vi "bylinear interpolation iiii- complex.vi"(0 "Array":cdb[](array[numeric]), 11 "center":i32=-1) -> (1 "radius":dbl, 2 "sigma":dbl, 3 "directed sigma - abs":dbl, 4 "left":cdb, 6 "center":cdb, 8 "right":cdb, 10 "directed sigma":cdb, 12 "intercept":cdb, 13 "slope":cdb, 14 "curvature":cdb, 15 "circle center":cdb)   [LabVIEW 2020]
uses:
  <vilib>/Analysis/baseanly.llb/Complex A x B.vi
  Q - not nan -- real.vi
  <vilib>/Analysis/Matrix/Numeric/Conversions/Array To Matrix.vi
  <vilib>/Analysis/Matrix/Numeric/Conversions/Array To Matrix - RA2.vi
  <vilib>/Analysis/baseanly.llb/Inverse Matrix.vi
  <vilib>/Analysis/baseanly.llb/Real Inverse Matrix.vi
  <vilib>/Analysis/NI_AALBase.lvlib
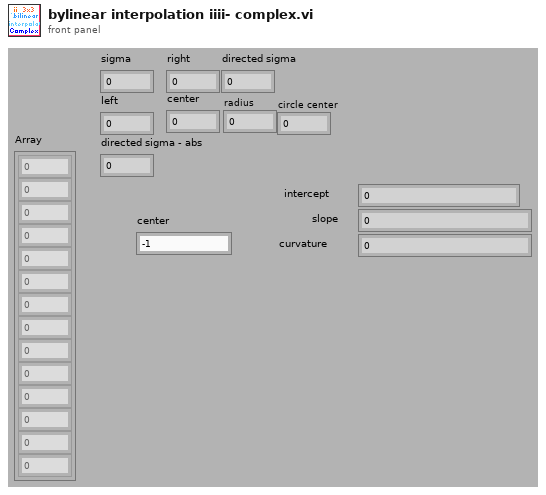
[diagram p1: front panel]
types:
  T1 = typedef "NI_Matrix.lvlib/RealMatrix.ctl" = dbl[][]
  T2 = typedef "NI_Matrix.lvlib/ComplexMatrix.ctl" = cdb[][]
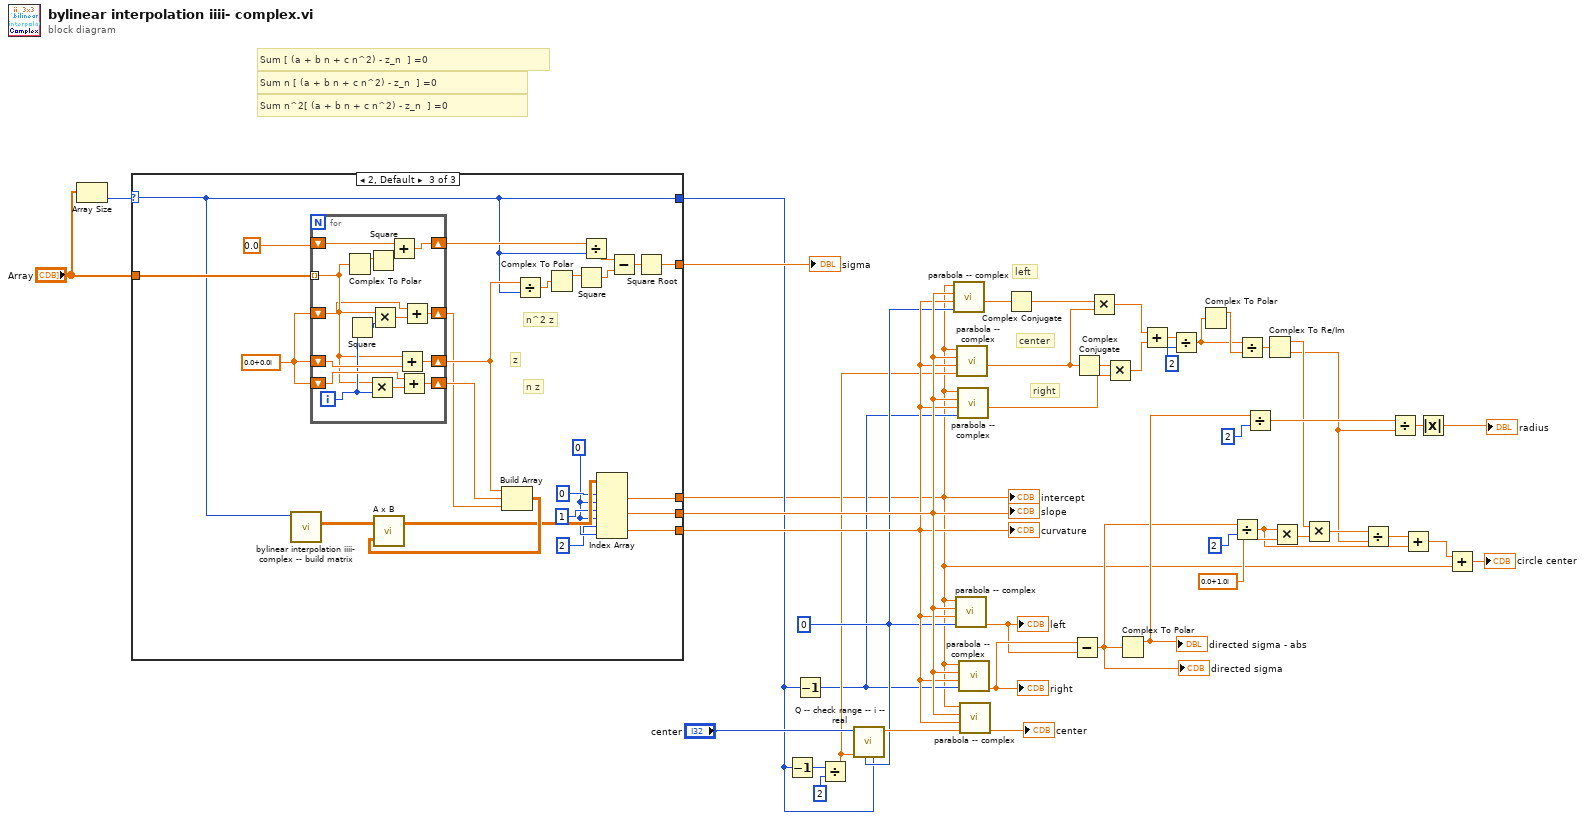
[diagram p0: block diagram]
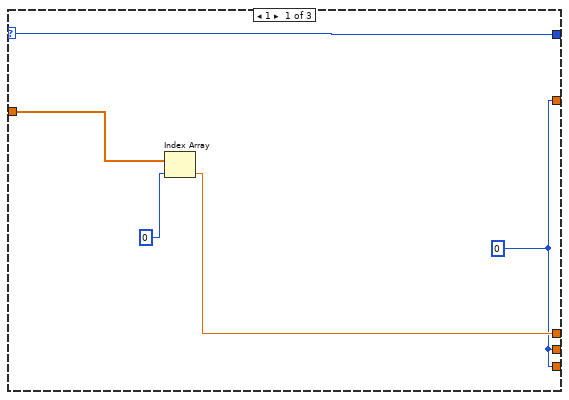
[diagram p2: hidden frame]
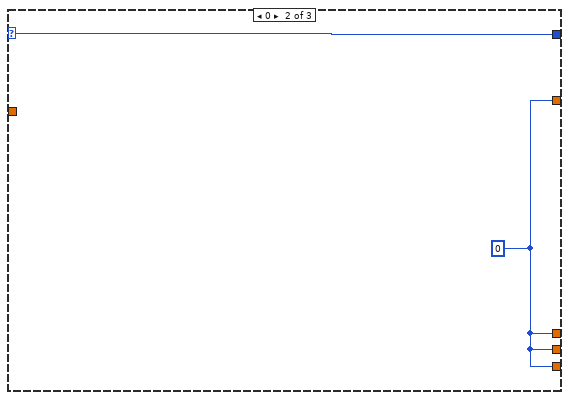
[diagram p3: hidden frame]
diagram:
  w35 = 0 ("n")
  # "right"
  # "center"
  # "left"
  # "Sum n^2[ (a + b n + c n^2) - z_n  ] =0"
  # "Sum n [ (a + b n + c n^2) - z_n  ] =0"
  # "Sum [ (a + b n + c n^2) - z_n  ] =0"
  n1 = Array Size(array="Array") -> (size(s)=w4:i32)
  n2 = case shown="2, Default" w4 {
    selector: w4 -> [w47 w52 w53]
    tunnel: [w48 w51 w56] -> w10
    tunnel: [w46 w51 w55] -> w37
    tunnel: "Array" -> [w50 _ w76]
    tunnel: [w46 w51 w75] -> w45
    tunnel: [w47 w52 w53] -> w33
    tunnel: [w46 w51 w54] -> w36
    frame 1 {
      w46 = 0 ("index")
      n3 = Index Array(array=w50, index=0) -> (element=w48:cdb)
    }
    frame 0 {
      w51 = 0 ("index")
    }
    frame 2, Default {
      w58 = 0 ("index (row)")
      w67 = cdb 0.0+0.0i
      # "n z"
      # "z"
      # "n^2 z"
      n4 = call "bylinear interpolation iiii- complex -- build matrix.vi"("N"=w53) -> ("Inverse Matrix"=w63:T1)  [unwired: 10 in]
      n5 = for {
        tunnel: w76 -> [w79] mode=indexing
        shift-right: [w91] -> w66
        shift-left: w67 -> [w90]
        shift-right: [w88] -> w65
        shift-left: w67 -> [w87]
        shift-right: [w86] -> w74
        shift-left: 0.0 -> [w85]
        shift-right: [w78] -> w64
        shift-left: w67 -> [w77]
        i -> [w82]
        n6 = Complex To Polar(r * e^(i*theta)=w79) -> (r=w84:dbl)  [unwired: 1 out]
        n7 = Square(x=w82) -> (x^2=w80:i32)
        n8 = Multiply(x=w79, y=w82) -> (x*y=w89:cdb)
        n9 = Square(x=w84) -> (x^2=w83:dbl)
        n10 = Multiply(x=w79, y=w80) -> (x*y=w81:cdb)
        n11 = Add(x=w85, y=w83) -> (x+y=w86:dbl)
        n12 = Add(x=w79, y=w90) -> (x+y=w91:cdb)
        n13 = Add(x=w87, y=w89) -> (x+y=w88:cdb)
        n14 = Add(x=w77, y=w81) -> (x+y=w78:cdb)
      }
      n15 = Build Array(w66, w65, w64) -> (w62:T2)
      n16 = call-poly <vilib>:"A x B.vi"("B"=w62, "A"=w63) -> ("A x B"=w61:T2)  [unwired: 1 out]
      n17 = Divide(x=w66, y=w53) -> (x/y=w71:cdb)
      n18 = Complex To Polar(r * e^(i*theta)=w71) -> (r=w72:dbl)  [unwired: 1 out]
      n19 = Square(x=w72) -> (x^2=w69:dbl)
      n20 = Divide(x=w74, y=w53) -> (x/y=w70:dbl)
      n21 = Index Array(array=w61, index (row) #1=0 ("index (row)"), index (col) #1=w58, index (row) #2=1 ("index (row)"), index (col) #2=w58, index (row) #3=2 ("index (row)"), index (col) #3=w58) -> (element #1=w56:cdb, element #2=w55:cdb, element #3=w54:cdb)
      n22 = Subtract(x=w70, y=w69) -> (x-y=w68:dbl)
      n23 = Square Root(x=w68) -> (sqrt(x)=w75:dbl)
    }
  }
  "slope" <- w37
  "intercept" <- w10
  "sigma" <- w45
  "curvature" <- w36
  n24 = Decrement(x=w33) -> (x-1=w44:i32)
  n25 = Decrement(x=w33) -> (x-1=w32:i32)
  n26 = Divide(x=w44, y=2 ("n")) -> (x/y=w34:dbl)
  n27 = call "Q -- check range -- i -- real.vi"("upper"=w33, "lower"=w35, "default"=w34, "number"="center") -> ("number in range"=w41:dbl)  [unwired: 5 in, 2 out]
  n28 = call "parabola -- complex.vi"("n"=w35, "curvature"=w36, "slope"=w37, "intercept"=w10) -> ("tangent"=w21:cdb)  [unwired: 6 in, 1 out]
  n29 = call "parabola -- complex.vi"("n"=w35, "curvature"=w36, "slope"=w37, "intercept"=w10) -> ("parabola"=w38:cdb)  [unwired: 6 in, 1 out]
  "left" <- w38
  n30 = call "parabola -- complex.vi"("n"=w34, "curvature"=w36, "slope"=w37, "intercept"=w10) -> ("tangent"=w19:cdb)  [unwired: 6 in, 1 out]
  n31 = call "parabola -- complex.vi"("n"=w32, "curvature"=w36, "slope"=w37, "intercept"=w10) -> ("tangent"=w3:cdb)  [unwired: 6 in, 1 out]
  n32 = call "parabola -- complex.vi"("n"=w32, "curvature"=w36, "slope"=w37, "intercept"=w10) -> ("parabola"=w39:cdb)  [unwired: 6 in, 1 out]
  "right" <- w39
  n33 = call "parabola -- complex.vi"("n"=w41, "curvature"=w36, "slope"=w37, "intercept"=w10) -> ("parabola"=→"center":cdb)  [unwired: 6 in, 1 out]
  n34 = Complex Conjugate(1:w21) -> (0:w20:cdb)
  n35 = Subtract(x=w39, y=w38) -> (x-y=w16:cdb)
  "directed sigma" <- w16
  n36 = Complex Conjugate(1:w19) -> (0:w18:cdb)
  n37 = Multiply(x=w20, y=w19) -> (x*y=w31:cdb)
  n38 = Multiply(x=w18, y=w3) -> (x*y=w30:cdb)
  n39 = Complex To Polar(r * e^(i*theta)=w16) -> (r=w25:dbl)  [unwired: 1 out]
  "directed sigma - abs" <- w25
  n40 = Add(x=w31, y=w30) -> (x+y=w29:cdb)
  n41 = Divide(x=w29, y=2) -> (x/y=w23:cdb)
  n42 = Complex To Polar(r * e^(i*theta)=w23) -> (r=w24:dbl)  [unwired: 1 out]
  n43 = Divide(x=w16, y=2) -> (x/y=w11:cdb)
  n44 = Divide(x=w23, y=w24) -> (x/y=w22:cdb)
  n45 = Divide(x=w25, y=2) -> (x/y=w26:dbl)
  n46 = Complex To Re/Im(x + iy=w22) -> (x=w2:dbl, y=w1:dbl)
  n47 = Multiply(x=w11, y=cdb 0.0+1.0i) -> (x*y=w14:cdb)
  n48 = Multiply(x=w2, y=w14) -> (x*y=w13:cdb)
  n49 = Divide(x=w13, y=w1) -> (x/y=w12:cdb)
  n50 = Divide(x=w26, y=w1) -> (x/y=w7:dbl)
  n51 = Add(x=w12, y=w11) -> (x+y=w9:cdb)
  n52 = Absolute Value(x=w7) -> (abs(x)=→"radius":dbl)
  n53 = Add(x=w9, y=w10) -> (x+y=→"circle center":cdb)
